vi "Create Panel Objects.vi"(8 "Error In":errorcluster, 11 "Pane Relief Main UI in":refnum<class "Pane Relief Main UI.lvclass">) -> (0 "Error Out":errorcluster, 3 "Pane Relief Main UI out":refnum<class "Pane Relief Main UI.lvclass">)   [LabVIEW 2015, in "Pane Relief Main UI.lvlib" / "Pane Relief Main UI.lvclass"]
uses:
  Pane Relief Main UI.lvclass
  Pane Relief Main UI.lvclass/Pane Relief Main UI.ctl
  Classes/Pane/Pane.lvclass
  Classes/Splitter/Splitter.lvclass
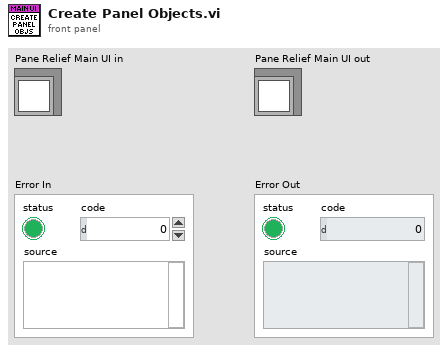
[diagram p1: front panel]
types:
  T1 = typedef "Selection Colors--Cluster.ctl" = cluster{"Normal":u32, "Mouse-over":u32, "Selected":u32, "Selected Mouse-over":u32}
  T2 = typedef "LVPointTypeDef.ctl" = cluster{"Horizontal":i16, "Vertical":i16}
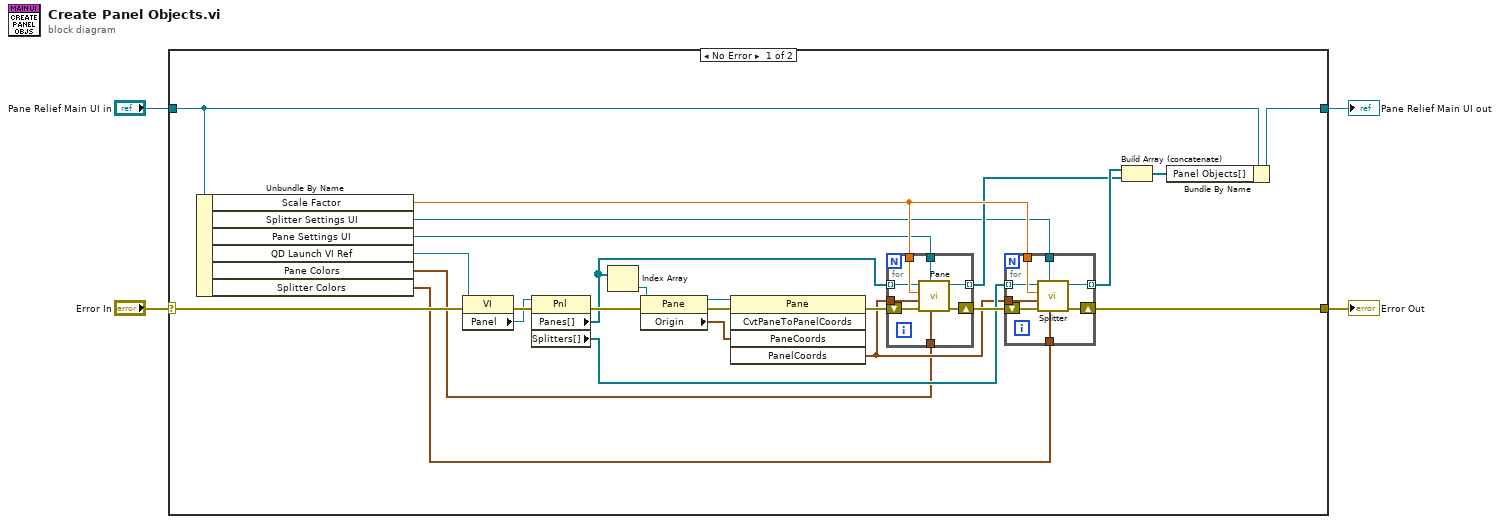
[diagram p0: block diagram]
diagram:
  n1 = case shown="No Error" "Error In" {
    selector: "Error In" -> [w9 w47]
    tunnel: [w8 w47] -> w1
    tunnel: [w13 w46] -> w3
    tunnel: "Pane Relief Main UI in" -> [w7 w46]
    frame No Error {
      n2 = Unbundle By Name(w7) -> ("Scale Factor"=w26:dbl, "Splitter Settings UI"=w11:refnum<class "Message Enqueuer.lvclass">, "Pane Settings UI"=w10:refnum<class "Message Enqueuer.lvclass">, "QD Launch VI Ref"=w12:refnum<vi>, "Pane Colors"=w6:T1, "Splitter Colors"=w5:T1)
      n3 = property class="VI"(reference=w12, error in=w9) -> (error out=w29:errorcluster, "Panel"=w28:refnum<vi>)  [unwired: 1 out]
      n4 = property class="Pnl"(reference=w28, error in=w29) -> (error out=w21:errorcluster, "Panes[]"=w16:refnum<vi>[], "Splitters[]"=w22:refnum<vi>[])  [unwired: 1 out]
      n5 = Index Array(array=w16) -> (element=w18:refnum<vi>)  [unwired: 1 in]
      n6 = property class="Pane"(reference=w18, error in=w21) -> (reference out=w25:refnum<vi>, error out=w24:errorcluster, "Origin"=w23:T2)
      n7 = invoke on="Invoke Node" class="Pane" method="CvtPaneToPanelCoords"(reference=w25, error in=w24, "PaneCoords"=w23) -> (error out=w20:errorcluster, "PanelCoords"=w19:T2)  [unwired: 2 in, 3 out]
      n8 = for {
        tunnel: w26 -> [w43]
        tunnel: w16 -> [w42] mode=indexing
        shift-right: [w44] -> w27
        shift-left: w20 -> [w45]
        tunnel: [w41] -> w14 mode=indexing
        tunnel: w19 -> [w40]
        tunnel: w10 -> [w39]
        tunnel: w6 -> [w38]
        n9 = call "Pane.vi"("Selection Colors"=w38, "Settings UI Enqueuer"=w39, "Error In"=w45, "Offset"=w40, "Scale Factor"=w43, "Pane Ref"=w42) -> ("Error Out"=w44:errorcluster, "Pane out"=w41:refnum<class "Pane.lvclass">)  [unwired: 4 in]
      }
      n10 = for {
        tunnel: w26 -> [w35]
        tunnel: w22 -> [w34] mode=indexing
        shift-right: [w37] -> w8
        shift-left: w27 -> [w36]
        tunnel: [w33] -> w15 mode=indexing
        tunnel: w19 -> [w32]
        tunnel: w11 -> [w31]
        tunnel: w5 -> [w30]
        n11 = call "Splitter.vi"("Selection Colors"=w30, "Settings UI Enqueuer"=w31, "Error In"=w36, "Offset"=w32, "Scale Factor"=w35, "Splitter Ref"=w34) -> ("Error Out"=w37:errorcluster, "Splitter out"=w33:refnum<class "Splitter.lvclass">)  [unwired: 4 in]
      }
      n12 = Build Array (concatenate)(w15, w14) -> (w17:refnum<class "Panel Object.lvclass">[])
      n13 = Bundle By Name(cluster=w7, "Panel Objects[]"=w17) -> (w13:refnum<class "Pane Relief Main UI.lvclass">)
    }
    frame Error {
    }
  }
  "Pane Relief Main UI out" <- w3
  "Error Out" <- w1
